vi "Basic Start Trigger.vi"(6 "ready for start trigger":bool=TRUE, 9 "data valid?":bool=TRUE, 10 "stream.state":T1, 11 "start trigger":bool=TRUE) -> (1 "data valid":bool=TRUE)   [LabVIEW 2015, in "niInstr Streaming v1 FPGA.lvlib"]
doc: "Provides a boolean start trigger function to control the start of data flow in a stream. All three boolean inputs are optional and default to True.\n\nA user should connect the Basic Start Trigger <b>stream.state</b> to the Data Stream Control <b>stream.state N</b> via a feedback node or shift register.\n\nWhen the stream enters a transferring state, it indicates that the stream is active, and therefore can activate the flow of data using the Basic Start Trigger.vi. The <b>data valid</b> output is gated on receiving a True on <b>start trigger</b> while the stream is active and <b>ready for start trigger</b> is also True. Once a start trigger is received, then the <B>data valid?</b> input is reflected through to the <b>data valid</b> output until the stream leaves an active state.\n\nThe <b>start trigger</b> does not need to coincide with a True on <B>data valid?</b> input."
uses:
  <instrlib>/_niInstr/Streaming/v1/FPGA/niInstr Streaming v1 FPGA.lvlib
  <instrlib>/_niInstr/Streaming/v1/Common/Stream State.ctl
  <instrlib>/_niInstr/Streaming/v1/Common/niInstr Streaming v1 Common.lvlib
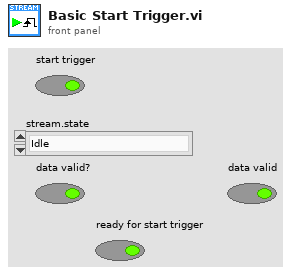
[diagram p1: front panel]
types:
  T1 = typedef "niInstr Streaming v1 Common.lvlib/Stream State.ctl" = enum8{"Idle", "Finite Transfer", "Continuous", "Done", "Error", "Not Ready", "Cancel"}
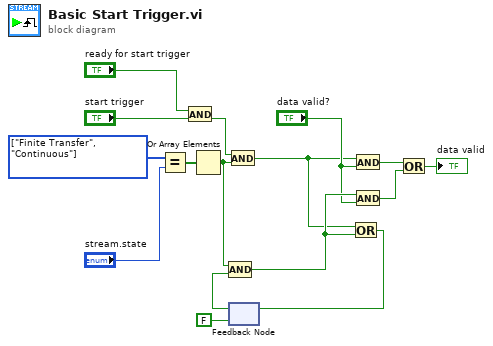
[diagram p0: block diagram]
diagram:
  w12 = T1[] [enum."Finite Transfer", enum."Continuous"] items=["Idle", "Finite Transfer", "Continuous", "Done", "Error", "Not Ready", "Cancel"]
  n1 = Equal?(x=w12, y="stream.state") -> (x = y?=w10:bool[])
  n2 = And(x="ready for start trigger", y="start trigger") -> (x .and. y?=w3:bool)
  n3 = Or Array Elements(Boolean array=w10) -> (logical OR=w1:bool)
  n4 = And(x=w3, y=w1) -> (x .and. y?=w4:bool)
  n5 = feedback #1(FALSE) -> (w9:bool)
  n6 = Compound Arithmetic op=AND(w1, w9) -> (w7:bool)
  n7 = Or(x=w4, y=w7) -> (x .or. y?=w8:bool)
  n8 = feedback-in #1(w8) -> ()
  n9 = And(x=w4, y="data valid?") -> (x .and. y?=w14:bool)
  n10 = And(x=w7, y="data valid?") -> (x .and. y?=w13:bool)
  n11 = Or(x=w14, y=w13) -> (x .or. y?=→"data valid":bool)
